vi "SetSerializableData_StaticCommunity.vi"(7 "BlueSerializer in":refnum<class "BlueSerializer.lvclass">, 8 "error in (no error)":errorcluster, 10 "Data In":T1={"StructuredData"=variant(string ""), "ClassOps (child, parent)"=[]}, 11 "BlueSerializable in":refnum<class "BlueSerializable.lvclass">) -> (0 "error out":errorcluster, 2 "Data Out":T1={"StructuredData"=variant(string ""), "ClassOps (child, parent)"=[]}, 3 "BlueSerializable out":refnum<class "BlueSerializable.lvclass">, 5 "BlueSerializer out":refnum<class "BlueSerializer.lvclass">)   [LabVIEW 2019, in "BlueSerialization.lvlib" / "BlueSerializable.lvclass"]
uses:
  BlueSerializable.lvclass
  BlueSerializer/BlueSerializer.lvclass
  BlueSerializer/Support/SetSerializableDataClusterLayer.ctl
  BlueSerializer/BlueSerializableVersion.ctl
  BlueSerializer/Support/SetSerializableDataClusterIterable.ctl
  BlueSerializer/Support/SetSerializableDataCluster.ctl
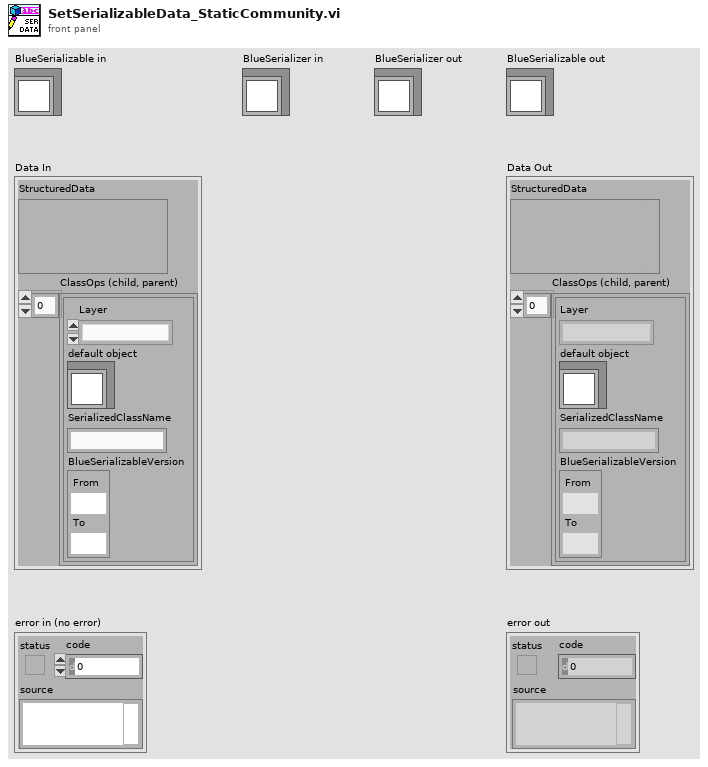
[diagram p1: front panel]
types:
  T1 = typedef "BlueSerialization.lvlib/BlueSerializer.lvclass/SetSerializableDataCluster.ctl" = cluster{"StructuredData":variant, "ClassOps (child, parent)":T2[]}
  T2 = typedef "BlueSerialization.lvlib/BlueSerializer.lvclass/SetSerializableDataClusterIterable.ctl" = cluster{"Layer":T3, "default object":refnum<class "BlueSerializable.lvclass">, "SerializedClassName":string, "BlueSerializableVersion":T4}
  T3 = typedef "BlueSerialization.lvlib/BlueSerializer.lvclass/SetSerializableDataClusterLayer.ctl" = enum16{"new class layer", "dropped class layer", "agreed class layer"}
  T4 = typedef "BlueSerialization.lvlib/BlueSerializer.lvclass/BlueSerializableVersion.ctl" = cluster{"From":u16, "To":u16}
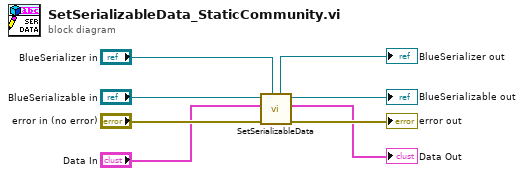
[diagram p0: block diagram]
diagram:
  n1 = call-dynamic "SetSerializableData.vi"("BlueSerializer in"="BlueSerializer in", "error in (no error)"="error in (no error)", "Data In"="Data In", "BlueSerializable in"="BlueSerializable in") -> ("error out"=→"error out":errorcluster, "Data Out"=→"Data Out":T1, "BlueSerializable out"=→"BlueSerializable out":refnum<class "BlueSerializable.lvclass">, "BlueSerializer out"=→"BlueSerializer out":refnum<class "BlueSerializer.lvclass">)  [unwired: 4 in]
